vi "SHAPE_SaveShapelets.vi"(8 "error in (no error)":errorcluster, 10 "Set of Shapelets":i32[][](array[numeric])=[[861, 12, 12], [22, 19, 11], [10, 1, 48], [448, 9, 27]], 11 "BandGlobalOpt in":refnum<class "Shapelets Search GA.lvclass">) -> (0 "error out":errorcluster, 2 "Class Label of Shapelet":string, 3 "BandGlobalOpt out":refnum<class "Shapelets Search GA.lvclass">)   [LabVIEW 2016, in "Shapelets Search (GA).lvlib" / "Shapelets Search GA.lvclass"]
uses:
  Shapelets Search GA.lvclass
  Shapelets Search GA.lvclass/Shapelets Search GA.ctl
  <vilib>/Analysis/baseanly.llb/Normalize Vector.vi
  <vilib>/Analysis/NI_AALBase.lvlib
panel:
  # "This VI is a part of BCI Design library, http://www.ru-bci.org \nCopyright © 2020, Sotnikov Peter, All rights reserved. License: CC BY-NC 4.0"
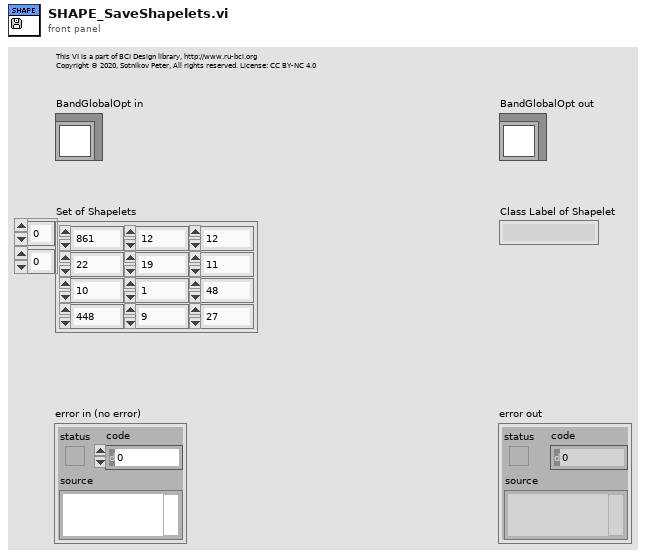
[diagram p1: front panel]
types:
  T1 = enum16{"big-endian, network order", "native, host order", "little-endian"}
  T2 = enum16{"open", "replace", "create", "open or create", "replace or create", "replace or create with confirmation"}
  T3 = typedef "Shapelets Search (GA).lvlib/SHAPE_SearchTypes.ctl" = enum16{"Лучший шейплет", "Набор шейплетов"}
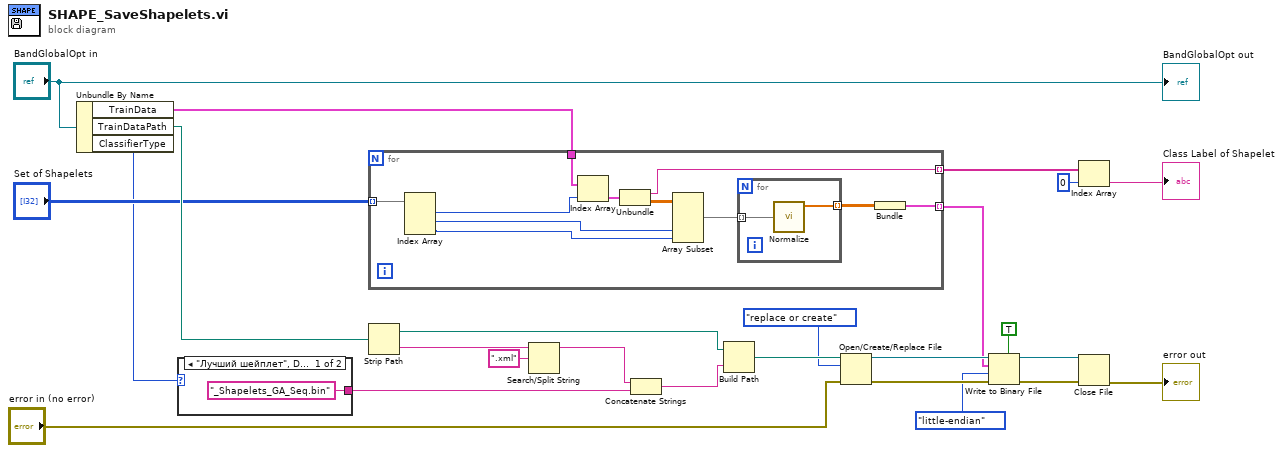
[diagram p0: block diagram]
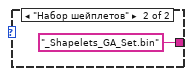
[diagram p2: hidden frame]
diagram:
  n1 = Unbundle By Name("BandGlobalOpt in") -> ("TrainData"=w9:cluster{"ClassLabel":string, "Trial":dbl[][]}[], "TrainDataPath"=w10:path, "ClassifierType"=w4:T3)
  n2 = case shown="\"Лучший шейплет\", Default" w4 {
    tunnel: ["_Shapelets_GA_Seq.bin" ("string") "_Shapelets_GA_Set.bin" ("string")] -> w22
    frame "Лучший шейплет", Default {
    }
    frame "Набор шейплетов" {
    }
  }
  n3 = for {
    tunnel: [w34] -> w14 mode=indexing
    tunnel: w9 -> [w33]
    tunnel: "Set of Shapelets" -> [w32] mode=indexing
    tunnel: [w28] -> w3 mode=indexing
    n4 = Index Array(array=w32) -> (element #1=w31:i32, element #2=w30:i32, element #3=w29:i32)  [unwired: 3 in]
    n5 = Index Array(array=w33, index=w31) -> (element=w38:cluster{"ClassLabel":string, "Trial":dbl[][]})
    n6 = Unbundle(w38) -> ("ClassLabel"=w28:string, "Trial"=w37:dbl[][])
    n7 = Array Subset(array=w37, index (col)=w30, length (col)=w29) -> (w36:dbl[][])  [unwired: 2 in]
    n8 = for {
      tunnel: [w40] -> w35 mode=indexing
      tunnel: w36 -> [w39] mode=indexing
      n9 = call-poly <vilib>:"Normalize.vi"("Vector"=w39) -> ("Normalized Vector"=w40:dbl[])  [unwired: 1 in, 3 out]
    }
    n10 = Bundle("Normalized Vector"=w35) -> (w34:cluster{"Normalized Vector":dbl[][]})  [unwired: 1 in]
  }
  n11 = Strip Path(path=w10) -> (stripped path=w21:path, name=w25:string)
  n12 = Search/Split String(string=w25, search string/char (-)=".xml") -> (substring before match=w23:string)  [unwired: 1 in, 2 out]
  n13 = Concatenate Strings(w23, w22) -> (w20:string)
  n14 = Build Path(base path=w21, name or relative path=w20) -> (appended path=w19:path)
  n15 = Open/Create/Replace File(file path (use dialog)=w19, error in="error in (no error)", operation (0:open)=T2."replace or create") -> (refnum out=w17:refnum<file>, error out=w16:errorcluster)  [unwired: 3 in, 1 out]
  n16 = Write to Binary File(file (use dialog)=w17, data=w14, error in=w16, 5:TRUE ("prepend array or string size? (T)"), 9:T1."little-endian" ("byte order (0:big-endian, network order)")) -> (refnum out=w12:refnum<file>, error out=w11:errorcluster)  [unwired: 1 in, 1 out]
  n17 = Index Array(array=w3, index=0) -> (element=→"Class Label of Shapelet":string)
  n18 = Close File(refnum=w12, error in=w11) -> (error out=→"error out":errorcluster)  [unwired: 1 out]
  "BandGlobalOpt out" <- "BandGlobalOpt in"
